vi "D2SParser - Private - Helper - Read Word.vi"(8 "error in (no error)":errorcluster, 10 "Position":i64, 11 "D2SParser in":refnum<class "D2SParser.lvclass">) -> (0 "error out":errorcluster, 2 "word":u16, 3 "D2SParser out":refnum<class "D2SParser.lvclass">)   [LabVIEW 2015, in "D2SParser.lvclass"]
uses:
  D2SParser.lvclass
  D2SParser.lvclass/D2SParser.ctl
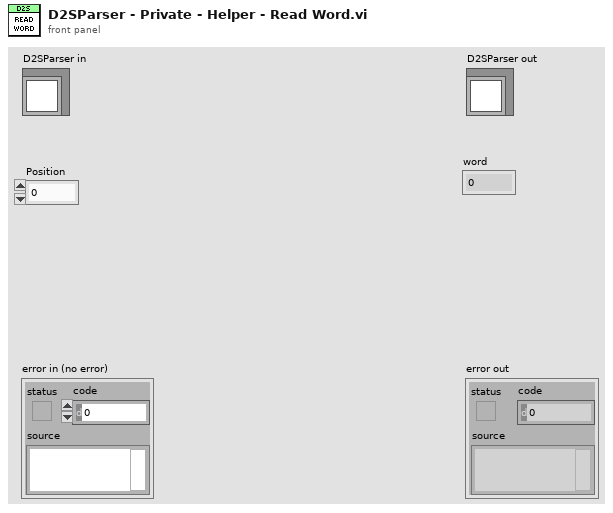
[diagram p1: front panel]
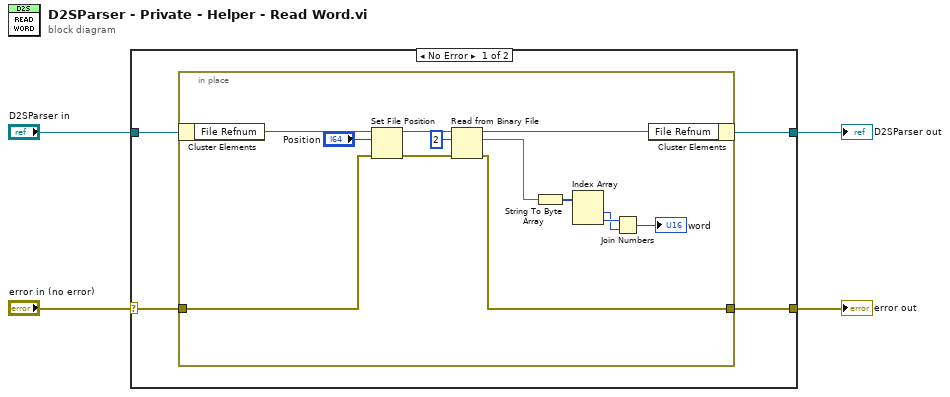
[diagram p0: block diagram]
diagram:
  n1 = case shown="No Error" "error in (no error)" {
    selector: "error in (no error)" -> [w7 w23]
    tunnel: [w6 w23] -> w3
    tunnel: [w5 w22] -> w1
    tunnel: "D2SParser in" -> [w8 w22]
    frame No Error {
      n2 = in-place {
        in-place-border: w7 -> [w16]
        in-place-border: [w13] -> w6
        n3 = in-place-cluster #1(w8) -> ("File Refnum"=w18:refnum<file>)
        n4 = Set File Position(offset (in bytes) (0)="Position", refnum=w18, error in=w16) -> (refnum out=w19:refnum<file>, error out=w20:errorcluster)  [unwired: 1 in]
        n5 = Read from Binary File(8:w20, 10:2 ("count (1)"), 11:w19) -> (0:w13:errorcluster, 2:w12:string, 3:w17:refnum<file>)  [unwired: 3 in, 1 out]
        n6 = String To Byte Array(string=w12) -> (unsigned byte array=w14:u8[])
        n7 = Index Array(array=w14) -> (element #1=w10:u8, element #2=w11:u8)  [unwired: 2 in]
        n8 = Join Numbers(hi=w11, lo=w10) -> ((hi.lo)=→"word":u16)
        n9 = in-place-cluster #1("File Refnum"=w17) -> (w5:refnum<class "D2SParser.lvclass">)
      }
    }
    frame Error {
    }
  }
  "error out" <- w3
  "D2SParser out" <- w1
